vi "Increment_Variables.vi"(8 "error in 2":errorcluster, 10 "Dummy Variable":dbl, 11 "Accelerometer":waveform(dbl)[](array[waveform])) -> (0 "error IO":errorcluster, 1 "X Accel Freq Array":dbl[](array[numeric]), 2 "Dummy Variable Array":dbl[](array[numeric]), 3 "Time Stamp":timestamp[](array[timestamp]), 4 "X Accel Mag Array":dbl[](array[numeric]), 5 "Y Accel Freq Array":dbl[](array[numeric]), 6 "Z Accel Freq Array":dbl[](array[numeric]), 7 "Y Accel Mag Array":dbl[](array[numeric]), 9 "Z Accel Mag Array":dbl[](array[numeric]))   [LabVIEW 2016]
uses:
  <vilib>/Utility/error.llb/DialogType.ctl
  <vilib>/express/express analysis/Spectral/Block/exnSpectralBlock spectral measurements RMS poly.vi
  <vilib>/express/express analysis/Spectral/Block/exnSpectralBlock spectral measurements RMS array WFM.vi
  <vilib>/express/express analysis/Spectral/XNode/ExpressSpectralMeasurementsBlockNode.xnode
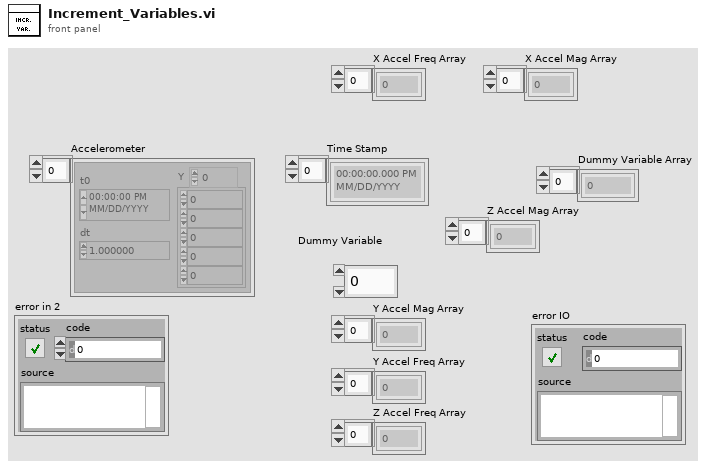
[diagram p1: front panel]
types:
  T1 = cluster{"averaging mode":u16, "weighting mode":u16, "number of averages":u32}
  T2 = cluster{"dB On (F)":bool, "unwrap phase (F)":bool, "convert to degree (F)":bool}
  T3 = typedef "DialogType.ctl" = u16
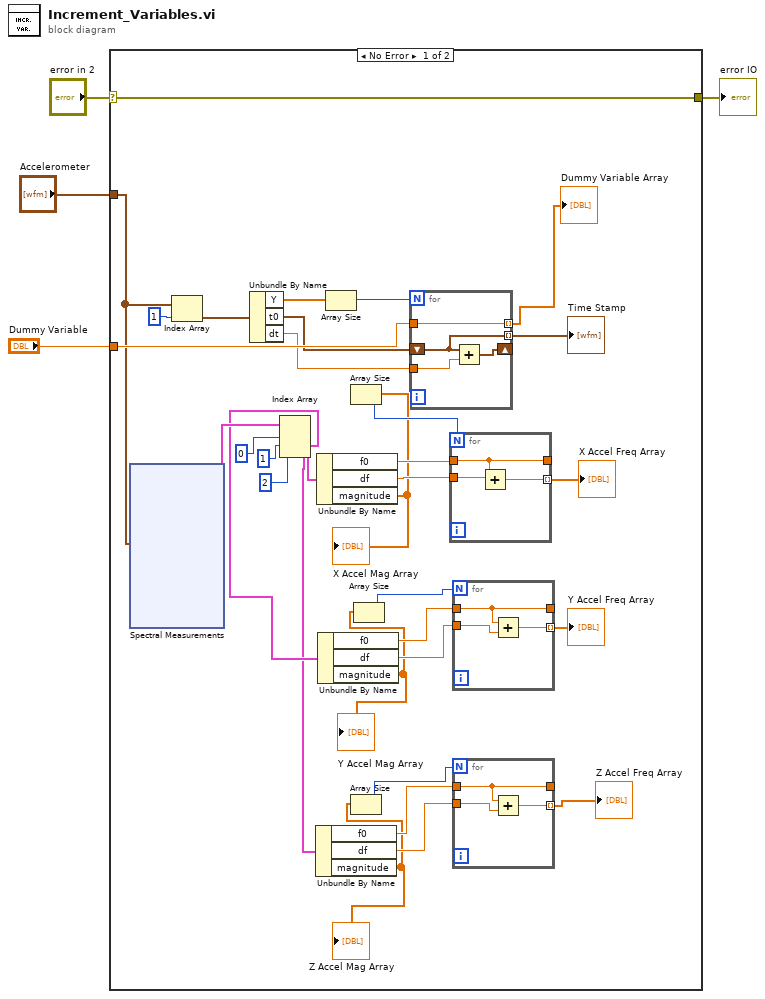
[diagram p0: block diagram]
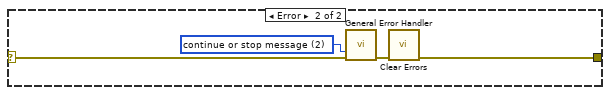
[diagram p2: hidden frame]
diagram:
  n1 = case shown="No Error" "error in 2" {
    selector: "error in 2" -> [w30 w62]
    tunnel: "Dummy Variable" -> [w37 _]
    tunnel: "Accelerometer" -> [w27 _]
    tunnel: [w30 w61] -> w2
    frame No Error {
      n2 = xnode "Spectral Measurements"("Signals"=w27) -> ("FFT - (RMS)"=w26:cluster{"f0":dbl, "df":dbl, "magnitude":dbl[]}[])  [unwired: 1 in, 2 out]
      n3 = Index Array(array=w27, index=1) -> (element=w35:waveform(dbl))
      n4 = Unbundle By Name(w35) -> ("Y"=w31:dbl[], "t0"=w33:timestamp, "dt"=w34:dbl)
      n5 = Index Array(array=w26, index #1=0 ("index"), index #2=1 ("index"), index #3=2 ("index")) -> (element #1=w24:cluster{"f0":dbl, "df":dbl, "magnitude":dbl[]}, element #2=w16:cluster{"f0":dbl, "df":dbl, "magnitude":dbl[]}, element #3=w15:cluster{"f0":dbl, "df":dbl, "magnitude":dbl[]})
      n6 = Unbundle By Name(w15) -> ("f0"=w8:dbl, "df"=w7:dbl, "magnitude"=w6:dbl[])
      "Z Accel Mag Array" <- w6
      n7 = Unbundle By Name(w24) -> ("f0"=w22:dbl, "df"=w21:dbl, "magnitude"=w19:dbl[])
      "X Accel Mag Array" <- w19
      n8 = Unbundle By Name(w16) -> ("f0"=w13:dbl, "df"=w12:dbl, "magnitude"=w10:dbl[])
      "Y Accel Mag Array" <- w10
      n9 = Array Size(array=w31) -> (size(s)=w32:i32)
      n10 = Array Size(array=w19) -> (size(s)=w23:i32)
      n11 = Array Size(array=w6) -> (size(s)=w9:i32)
      n12 = Array Size(array=w10) -> (size(s)=w14:i32)
      n13 = for {
        N: w32 -> [_]
        tunnel: w34 -> [w60]
        shift-right: [w59] -> _
        shift-left: w33 -> [w58]
        tunnel: [w58] -> w28 mode=indexing
        tunnel: [w57] -> w29 mode=indexing
        tunnel: w37 -> [w57]
        n14 = Add(x=w58, y=w60) -> (x+y=w59:timestamp)
      }
      "Time Stamp" <- w28
      "Dummy Variable Array" <- w29
      n15 = for {
        N: w23 -> [_]
        tunnel: w21 -> [w46]
        tunnel: [w45] -> w20 mode=indexing
        tunnel: w22 -> [w44]
        tunnel: [w44] -> _
        n16 = Add(x=w44, y=w46) -> (x+y=w45:dbl)
      }
      "X Accel Freq Array" <- w20
      n17 = for {
        N: w14 -> [_]
        tunnel: w12 -> [w43]
        tunnel: [w42] -> w11 mode=indexing
        tunnel: w13 -> [w41]
        tunnel: [w41] -> _
        n18 = Add(x=w41, y=w43) -> (x+y=w42:dbl)
      }
      "Y Accel Freq Array" <- w11
      n19 = for {
        N: w9 -> [_]
        tunnel: w7 -> [w40]
        tunnel: [w39] -> w5 mode=indexing
        tunnel: w8 -> [w38]
        tunnel: [w38] -> _
        n20 = Add(x=w38, y=w40) -> (x+y=w39:dbl)
      }
      "Z Accel Freq Array" <- w5
    }
    frame Error {
      w63 = T3 2 items=["no dialog", "OK message", "continue or stop message", "OK message + warnings", "continue/stop + warnings"] ("type of dialog (OK msg:1)")
      n21 = call <vilib>:"General Error Handler.vi"("type of dialog (OK msg:1)"=w63, "error in (no error)"=w62) -> ("error out"=w64:errorcluster)  [unwired: 9 in, 4 out]
      n22 = call <vilib>:"Clear Errors.vi"("error in (no error)"=w64) -> ("error out"=w61:errorcluster)  [unwired: 5 in, 1 out]
    }
  }
  "error IO" <- w2
